vi "Outer Condition.vi"(8 "error in (no error)":errorcluster, 11 "Measurement3D in":refnum<class "Measurement3D.lvclass">) -> (0 "error out":errorcluster, 2 "Finish?":bool, 3 "Measurement3D out":refnum<class "Measurement3D.lvclass">)   [LabVIEW 2014, in "Measurement3D.lvclass"]
uses:
  Measurement3D.lvclass
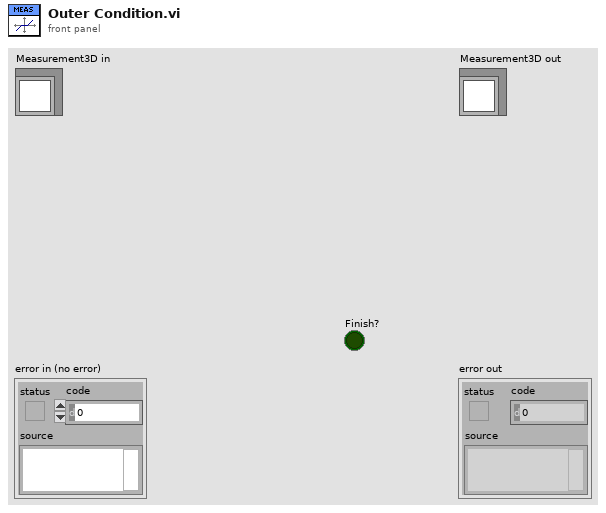
[diagram p1: front panel]
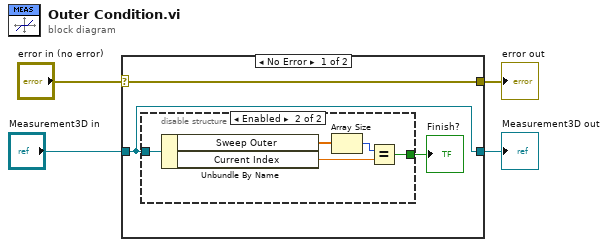
[diagram p0: block diagram]
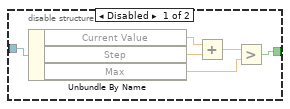
[diagram p2: hidden frame]
diagram:
  n1 = case shown="No Error" "error in (no error)" {
    selector: "error in (no error)" -> [w7 w20]
    tunnel: [w7 w20] -> w3
    tunnel: [w6 w19] -> w1
    tunnel: "Measurement3D in" -> [w6 w19]
    frame No Error {
      n2 = disable-structure shown="Enabled" {
        disable-tunnel: w6 -> [w12 w18]
        disable-tunnel: [w8 w14] -> w5
        frame Disabled {
          n3 = Unbundle By Name(w12) -> ("Current Value"=w11:dbl, "Step"=w10:dbl, "Max"=w9:dbl)
          n4 = Add(x=w11, y=w10) -> (x+y=w13:dbl)
          n5 = Greater?(x=w13, y=w9) -> (0:w8:bool)
        }
        frame Enabled {
          n6 = Unbundle By Name(w18) -> ("Sweep Outer"=w17:dbl[], "Current Index"=w15:dbl)
          n7 = Array Size(array=w17) -> (size(s)=w16:i32)
          n8 = Equal?(x=w16, y=w15) -> (x = y?=w14:bool)
        }
      }
      "Finish?" <- w5
    }
    frame Error {
    }
  }
  "error out" <- w3
  "Measurement3D out" <- w1
